vi "Read CSV worksheet.vi"(8 "error in (no error)":errorcluster, 11 "appended path":path) -> (0 "error out":errorcluster, 3 "Sheet":string[][](array[string]))   [LabVIEW 2026, in "TALOS.lvlib"]
doc: "This VI is used to open a CSV and output a matrix of strings out of it."
uses:
  TALOS.lvlib
  <vilib>/Utility/file.llb/Read Delimited Spreadsheet (string).vi
panel:
  in  "worksheet index":i32
  # "No more used"
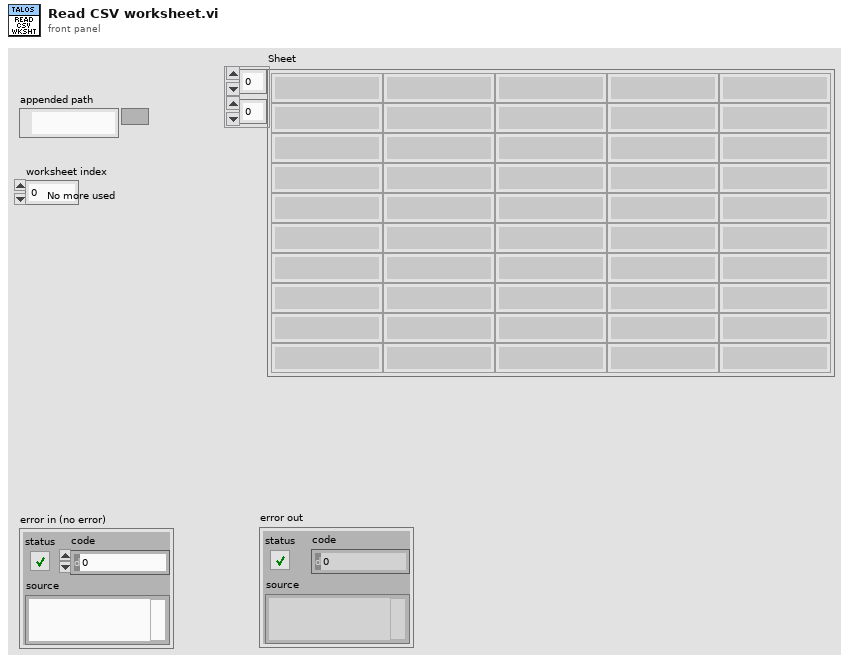
[diagram p1: front panel]
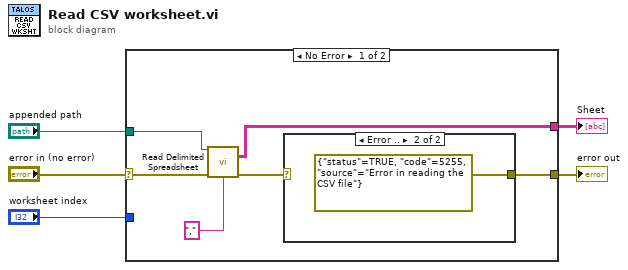
[diagram p0: block diagram]
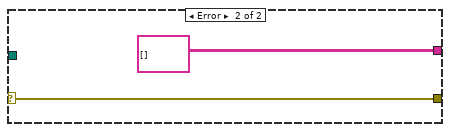
[diagram p3: hidden frame]
diagram:
  n1 = case shown="No Error" "error in (no error)" {
    selector: "error in (no error)" -> [w10 w14]
    tunnel: "worksheet index" -> [_ _]
    tunnel: [w11 string[][] [] ("data")] -> w4
    tunnel: "appended path" -> [w9 _]
    tunnel: [w6 w14] -> w1
    frame No Error {
      n2 = call-poly <vilib>:"Read Delimited Spreadsheet.vi"("file path (dialog if empty)"=w9, "error in (no error)"=w10, "delimiter (\\t)"="," ("delimiter (\\t)")) -> ("all rows"=w11:string[][], "error out"=w7:errorcluster)  [unwired: 7 in, 4 out]
      n3 = case shown="Error .." w7 {
        selector: w7 -> [w12 _]
        tunnel: [w12 errorcluster {"status"=TRUE, "code"=5255, "source"="Error in reading the CSV file"} ("error in")] -> w6
        frame No Error {
        }
        frame Error {
        }
      }
    }
    frame Error {
    }
  }
  "Sheet" <- w4
  "error out" <- w1
